vi "InitH5.vi"(7 "Attributes":T1={"ChName"="CH1", "\nCoupling"=1, "RangeV"=1.0, "OffsetV"=-0.45, "InputImpedanceOhms"="FIFTY", "TimePerRecordSec"=2e-06, "AcqStartTimeSec"=-5e-07, "TickTimeSecs"=0.0, "TriggerSource"="CH1", "TriggerSlope"=1, "TrigLevelV"=-0.1} {"Coupling" items=["AC", "DC", "GND"]; "TriggerSlope" items=["Positive", "Negative"]}, 8 "error in (no error)":errorcluster, 10 "String":string, 11 "base path":path) -> (0 "error out":errorcluster, 2 "HDF5 Dataset Ref out":T2, 3 "Refnum out":T2)   [LabVIEW 2011]
uses:
  <vilib>/UPVI/lvhdf5/library.llb/HDF5 Ref.ctl
  <vilib>/UPVI/lvhdf5/dataset.llb/LVH5D Operation.ctl
  <vilib>/UPVI/lvhdf5/attribute.llb/LVH5A Operation.ctl
  <vilib>/UPVI/lvhdf5/dataset.llb/Simple OpenCreateReplace Dataset (Variant).vi
  <vilib>/UPVI/lvhdf5/attribute.llb/Write Multiple Attributes.vi
  <vilib>/Utility/VariantDataType/GetClusterInfo.vi
  <vilib>/Utility/VariantDataType/GetTypeInfo.vi
  <vilib>/UPVI/lvhdf5/dataset.llb/Simple OpenCreateReplace Dataset.xnode
  <vilib>/UPVI/lvhdf5/attribute.llb/LVH5 Write Attributes.xnode
  <vilib>/UPVI/lvhdf5/attribute.llb/Cluster to Attribute Array.xnode
  <vilib>/Utility/VariantDataType/VariantType.lvlib
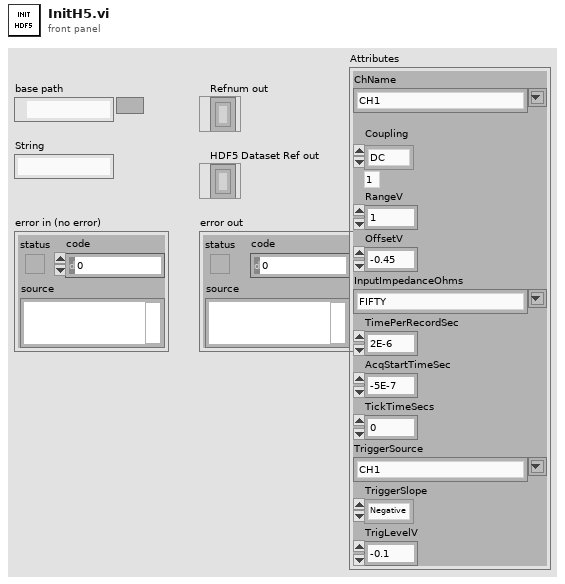
[diagram p1: front panel]
types:
  T1 = cluster{"ChName":string, "\nCoupling":i32, "RangeV":dbl, "OffsetV":dbl, "InputImpedanceOhms":string, "TimePerRecordSec":dbl, "AcqStartTimeSec":dbl, "TickTimeSecs":dbl, "TriggerSource":string, "TriggerSlope":i32, "TrigLevelV":dbl}
  T2 = typedef "HDF5 Ref.ctl" = refnum<k1>
  T3 = typedef "LVH5A Operation.ctl" = enum16{"open", "replace", "create", "open or create", "create or replace", "create or replace with confirmation"}
  T4 = typedef "LVH5D Operation.ctl" = enum16{"open", "replace", "create", "open or create", "create or replace", "create or replace with confirmation"}
  T5 = cluster{"Voltage":dbl[], "StartTime":timestamp}[]
  T6 = cluster{"Voltage":dbl[], "StartTime":timestamp}[][]
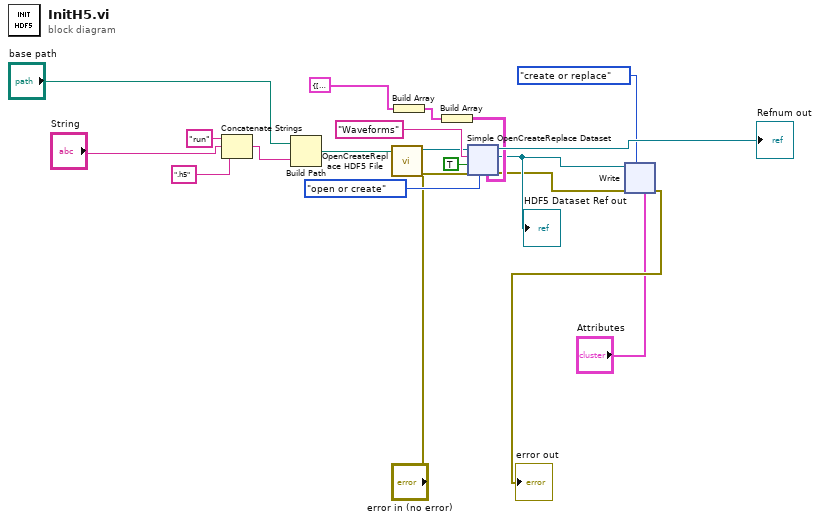
[diagram p0: block diagram]
diagram:
  n1 = Concatenate Strings("run" ("string"), "String", ".h5" ("string")) -> (w9:string)
  n2 = Build Path(base path="base path", name or relative path=w9) -> (appended path=w11:path)
  n3 = call <vilib>:"OpenCreateReplace HDF5 File.vi"("error in (no error)"="error in (no error)", "path"=w11) -> ("error out"=w14:errorcluster, "HDF5 Ref out"=w13:T2)  [unwired: 6 in]
  n4 = Build Array(cluster{"Voltage":dbl[], "StartTime":timestamp} {"Voltage"=[], "StartTime"=timestamp(0 s since 1904-01-01)}) -> (w19:T5)
  n5 = Build Array(w19) -> (w20:T6)
  n6 = xnode "Simple OpenCreateReplace Dataset"("Dataset Path"="Waveforms", "HDF5 Ref"=w13, "Unlimited  dataset (F)"=TRUE, "error in (no error)"=w14, "operation"=LVH5D_Operation."open or create" ("operation (open or create)"), "Datatype and Dataspace"=w20) -> ("HDF5 Dataset Ref out"=w4:T2, "HDF5 Ref out"=→"Refnum out":T2, "error out"=w3:errorcluster)  [unwired: 2 in]
  "HDF5 Dataset Ref out" <- w4
  n7 = xnode "Write"("HDF5 Ref"=w4, "error in (no error)"=w3, "operation (create or replace)"=LVH5A_Operation."create or replace", "Value(s)"="Attributes") -> ("error out"=→"error out":errorcluster)  [unwired: 1 in, 1 out]
